vi "List Shared Resources.vi"(8 "error in (no error)":errorcluster) -> (0 "error out":errorcluster, 2 "Shared Resources":refnum<class "SMO.lvclass">[](array[class]))   [LabVIEW 2019, in "Registry-SMO.lvclass"]
doc: "JKI State Machine Objects (SMO) 1.3.0.56\nJKI - JKI\nCopyright (c) 2017, JKI"
uses:
  Registry-SMO.lvclass
  SMO/SMO.lvclass
  Registry-SMO.lvclass/Registry-SMO.ctl
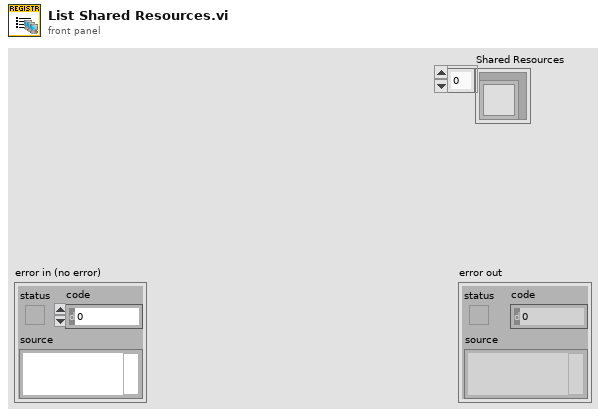
[diagram p1: front panel]
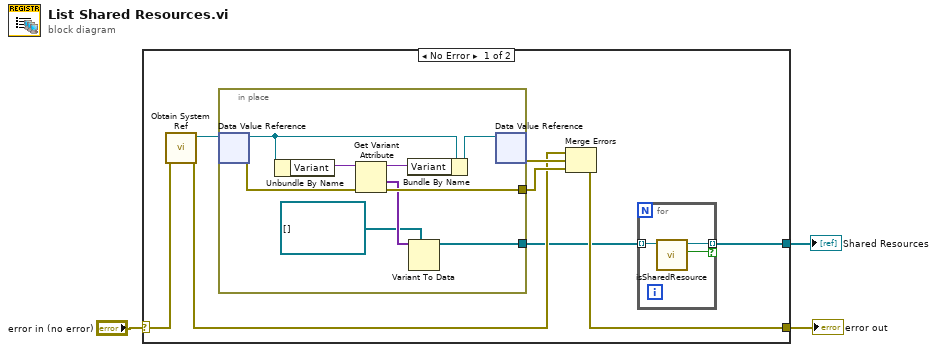
[diagram p0: block diagram]
diagram:
  n1 = case shown="No Error" "error in (no error)" {
    selector: "error in (no error)" -> [w8 w24]
    tunnel: [w6 w24] -> w2
    tunnel: [w4 _] -> w1
    frame No Error {
      n2 = call "Obtain System Ref.vi"("error in (no error)"=w8) -> ("error out"=w7:errorcluster, "JKI SMO System"=w9:refnum<data-value>)  [unwired: 9 in]
      n3 = in-place {
        in-place-border: [w18] -> w10
        in-place-border: [w15] -> w5
        n4 = in-place-dvr #1(w9) -> (w23:refnum<class "Registry-SMO.lvclass">, w19:errorcluster)
        n5 = Unbundle By Name(w23) -> ("Variant"=w21:variant)
        n6 = Get Variant Attribute(Variant=w21, error in=w19) -> (duplicate Variant=w20:variant, values=w17:variant[], error out=w18:errorcluster)  [unwired: 2 in, 1 out]
        n7 = Bundle By Name(cluster=w23, "Variant"=w20) -> (w22:refnum<class "Registry-SMO.lvclass">)
        n8 = Variant To Data(type=refnum<class "SMO.lvclass">[] [], Variant=w17) -> (data=w15:refnum<class "SMO.lvclass">[])  [unwired: 1 in, 1 out]
        n9 = in-place-dvr #1(w22) -> (w11:errorcluster)  [unwired: 1 out]
      }
      n10 = Merge Errors(w7, w11, w10) -> (w6:errorcluster)
      n11 = for {
        tunnel: w5 -> [w14] mode=indexing
        tunnel: [w13] -> w4 mode=indexing if=w12
        n12 = call "isSharedResource.vi"("SMO in"=w14) -> ("shared resource"=w12:bool, "SMO out"=w13:refnum<class "SMO.lvclass">)  [unwired: 8 in, 1 out]
      }
    }
    frame Error {
    }
  }
  "error out" <- w2
  "Shared Resources" <- w1
